vi "Build Sensor Visualisation.vi"(1 "Sensors":map{T2, T3}(c390)) -> (0 "Sensor Coverage Visualisation":T1(array[cluster]))   [LabVIEW 2020, in "AoC 2022.lvlib"]
uses:
  AoC 2022.lvlib
  Location.ctl
  Coverage Area.ctl
  Sensor Info.ctl
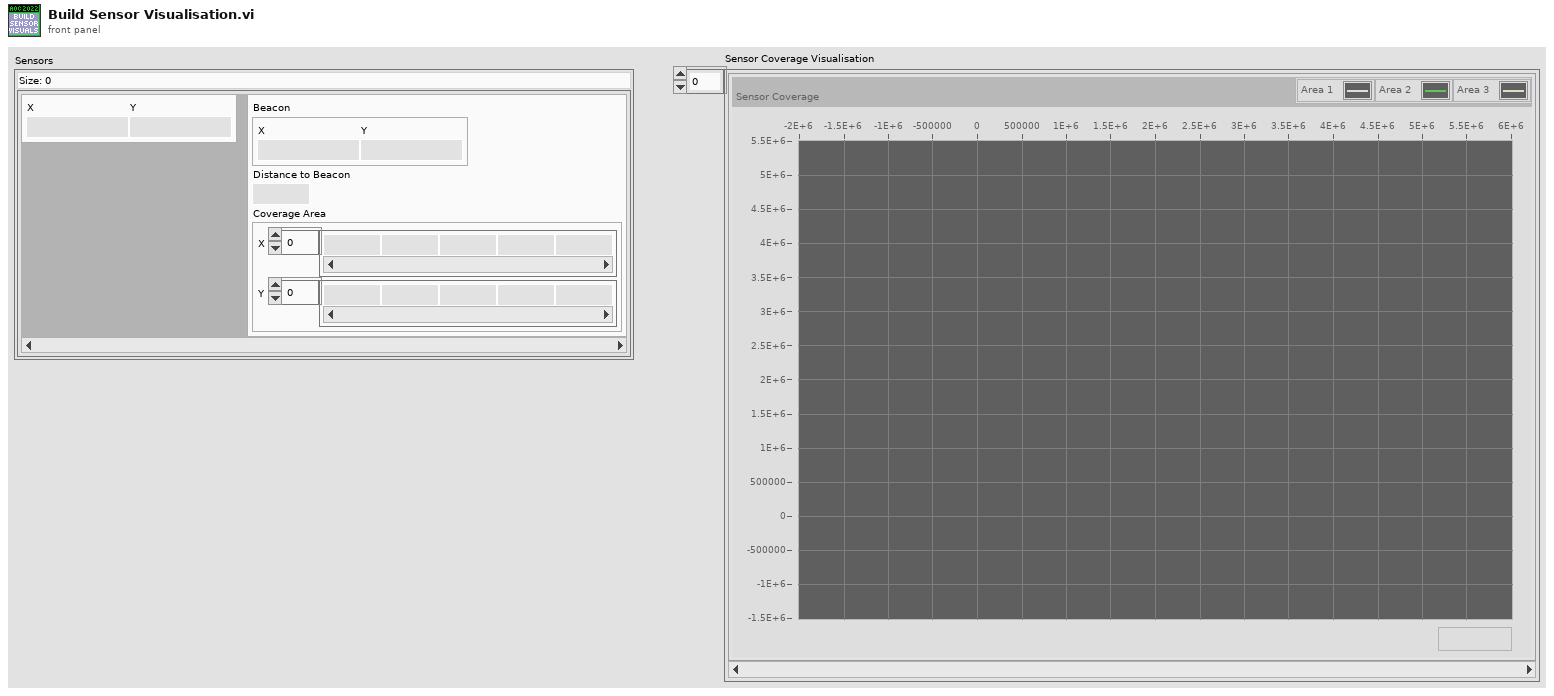
[diagram p1: front panel]
types:
  T1 = cluster{"Sensor Coverage":cluster{cluster{"X":dbl, "Y":dbl}[]}[]}[]
  T2 = typedef "AoC 2022.lvlib/Location.ctl" = cluster{"X":i32, "Y":i32}
  T3 = typedef "AoC 2022.lvlib/Sensor Info.ctl" = cluster{"Beacon":T2, "Distance to Beacon":dbl, "Coverage Area":T4}
  T4 = typedef "AoC 2022.lvlib/Coverage Area.ctl" = cluster{"X":dbl[], "Y":dbl[]}
  T5 = cluster{"Points":cluster{"X":dbl, "Y":dbl}[], "Hole":bool}[]
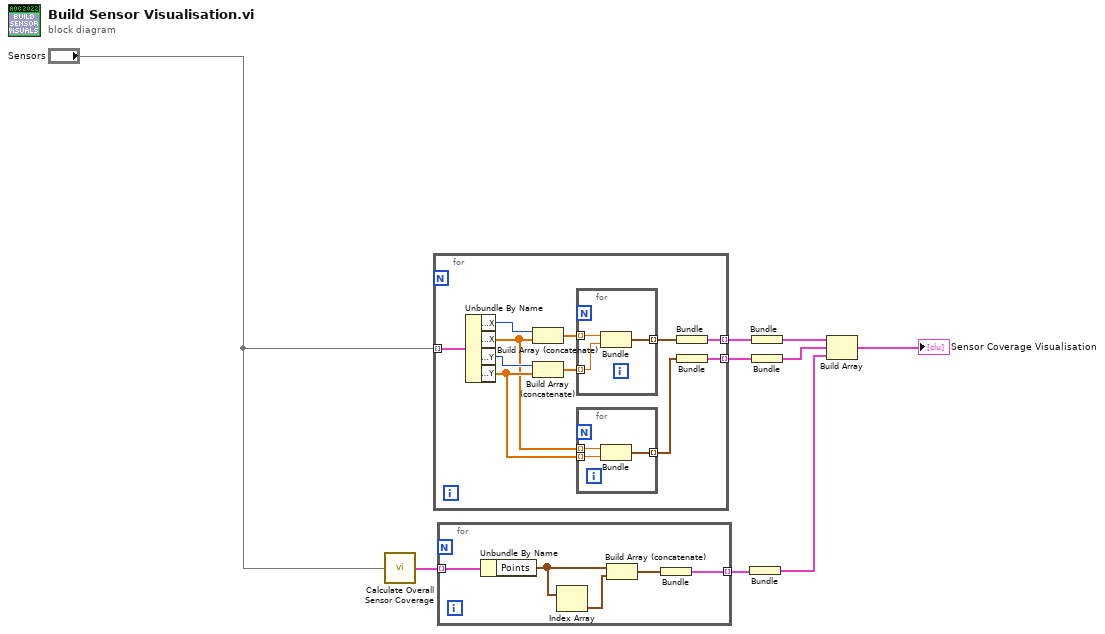
[diagram p0: block diagram]
diagram:
  n1 = call "Calculate Overall Sensor Coverage.vi"("Sensors"="Sensors") -> ("Overall Sensor Coverage"=w9:T5)
  n2 = for {
    tunnel: "Sensors" -> [w20] mode=indexing
    tunnel: [w14] -> w2 mode=indexing
    tunnel: [w13] -> w5 mode=indexing
    n3 = Unbundle By Name(w20) -> ("Sensor.X"=w19:i32, "Sensor Info.Coverage Area.X"=w11:dbl[], "Sensor.Y"=w18:i32, "Sensor Info.Coverage Area.Y"=w12:dbl[])
    n4 = Build Array (concatenate)(w19, w11) -> (w17:dbl[])
    n5 = Build Array (concatenate)(w18, w12) -> (w16:dbl[])
    n6 = for {
      tunnel: w17 -> [w23] mode=indexing
      tunnel: w16 -> [w22] mode=indexing
      tunnel: [w21] -> w15 mode=indexing
      n7 = Bundle("X"=w23, "Y"=w22) -> (w21:cluster{"X":dbl, "Y":dbl})  [unwired: 1 in]
    }
    n8 = for {
      tunnel: w11 -> [w26] mode=indexing
      tunnel: [w25] -> w10 mode=indexing
      tunnel: w12 -> [w24] mode=indexing
      n9 = Bundle("X"=w26, "Y"=w24) -> (w25:cluster{"X":dbl, "Y":dbl})  [unwired: 1 in]
    }
    n10 = Bundle(w15) -> (w14:cluster{cluster{"X":dbl, "Y":dbl}[]})  [unwired: 1 in]
    n11 = Bundle(w10) -> (w13:cluster{cluster{"X":dbl, "Y":dbl}[]})  [unwired: 1 in]
  }
  n12 = for {
    tunnel: w9 -> [w31] mode=indexing
    tunnel: [w28] -> w1 mode=indexing
    n13 = Unbundle By Name(w31) -> ("Points"=w30:cluster{"X":dbl, "Y":dbl}[])
    n14 = Index Array(array=w30) -> (element=w27:cluster{"X":dbl, "Y":dbl})  [unwired: 1 in]
    n15 = Build Array (concatenate)(w30, w27) -> (w29:cluster{"X":dbl, "Y":dbl}[])
    n16 = Bundle(w29) -> (w28:cluster{cluster{"X":dbl, "Y":dbl}[]})  [unwired: 1 in]
  }
  n17 = Bundle(w1) -> (w7:cluster{cluster{cluster[]}[]})  [unwired: 1 in]
  n18 = Bundle(w2) -> (w3:cluster{cluster{cluster[]}[]})  [unwired: 1 in]
  n19 = Bundle(w5) -> (w6:cluster{cluster{cluster[]}[]})  [unwired: 1 in]
  n20 = Build Array(w3, w6, w7) -> (→"Sensor Coverage Visualisation":cluster{cluster{cluster[]}[]}[])
